vi "HFRR ADV v04.vi"() -> ()   [LabVIEW 2025] (continued)
        n290 = event-data() -> ()  [unwired: 1 in, 6 out]
        n291 = local read "Headen Service Button"() -> (w388:bool)
        n292 = case shown="True" w388 {
          frame False {
            n293 = property on="Password 3" class="Clust (strict)"("Visible"=FALSE) -> ()  [unwired: 2 in, 2 out]
            n294 = property on="Service Password Log" class="Str"("Visible"=FALSE) -> ()  [unwired: 2 in, 2 out]
          }
          frame True {
            n295 = property on="Password 3" class="Clust (strict)"("Visible"=TRUE) -> ()  [unwired: 2 in, 2 out]
            n296 = property on="Service Password Log" class="Str"("Visible"=TRUE) -> ()  [unwired: 2 in, 2 out]
          }
        }
      }
      event "Password 3.Service Password": Value Change {
        n297 = event-data() -> ()  [unwired: 1 in, 6 out]
        n298 = Unbundle By Name("Password 3") -> ("Service Password"=w395:string)
        n299 = call <vilib>:"Trim Whitespace.vi"("string"=w395) -> ("trimmed string"=w393:string)  [unwired: 1 in]
        n300 = Equal?(x=w393, y="Service@123") -> (x = y?=w394:bool)
        n301 = case shown="False" w394 {
          selector: w394 -> [w399 w401]
          frame False {
            n302 = local write "Service Password enable"(w399) -> ()
            n303 = property on="Service Password Log" class="Str"("Visible"=TRUE) -> ()  [unwired: 2 in, 2 out]
            n304 = property on="Tab Control 5" class="TabCtl (strict)"("Tabs Visible?"=TRUE ("Page Labels Display Visible?")) -> ()  [unwired: 2 in, 2 out]
          }
          frame True {
            n305 = property on="Service Password Log" class="Str"("Visible"=FALSE) -> ()  [unwired: 2 in, 2 out]
            "Service Password enable" <- w401
          }
        }
      }
      event "Sign In": Value Change {
        w403 = FALSE ("Visible")
        n306 = event-data() -> ()  [unwired: 1 in, 6 out]
        n307 = property on="About" class="Clust (strict)"("Visible"=w403) -> ()  [unwired: 2 in, 2 out]
        n308 = property on="Password 3" class="Clust (strict)"("Visible"=w403) -> ()  [unwired: 2 in, 2 out]
        n309 = property on="Service Password Log" class="Str"("Visible"=FALSE) -> ()  [unwired: 2 in, 2 out]
      }
      event "Info": Value Change {
        n310 = event-data() -> ()  [unwired: 1 in, 6 out]
        n311 = local read "Info"() -> (w405:bool)
        n312 = case shown="False" w405 {
          frame False {
            n313 = property on="About" class="Clust (strict)"("Visible"=FALSE) -> ()  [unwired: 2 in, 2 out]
          }
          frame True {
            n314 = property on="About" class="Clust (strict)"("Visible"=TRUE) -> ()  [unwired: 2 in, 2 out]
          }
        }
      }
      event "Calibration": Value Change {
        n315 = event-data() -> ()  [unwired: 1 in, 6 out]
        n316 = local read "Calibration"() -> (w409:bool)
        n317 = case shown="False" w409 {
          frame False {
            n318 = property on="Calibration 2" class="TabCtl (strict)"("Visible"=FALSE) -> ()  [unwired: 2 in, 2 out]
            n319 = local write "Cal Password"("" ("Cal Password")) -> ()
          }
          frame True {
            n320 = property on="Calibration 2" class="TabCtl (strict)"("Visible"=TRUE) -> ()  [unwired: 2 in, 2 out]
            n321 = local write "Cal Password"("" ("Cal Password")) -> ()
          }
        }
        n322 = property on="Wrong Password" class="Str"("Visible"=FALSE) -> ()  [unwired: 2 in, 2 out]
      }
      event "Cal Password": Value Change {
        n323 = event-data() -> ()  [unwired: 1 in, 6 out]
        n324 = local read "Cal Password"() -> (w417:string)
        n325 = call <vilib>:"Trim Whitespace.vi"("string"=w417) -> ("trimmed string"=w416:string)  [unwired: 1 in]
        n326 = Equal?(x=w416, y="Cal@321") -> (x = y?=w414:bool)
        n327 = case shown="True" w414 {
          frame False {
            n328 = property on="Wrong Password" class="Str"("Visible"=TRUE) -> ()  [unwired: 2 in, 2 out]
          }
          frame True {
            n329 = property on="Wrong Password" class="Str"("Visible"=FALSE) -> ()  [unwired: 2 in, 2 out]
            n330 = local write "Main Tab"(T2."About" ("Main Tab")) -> ()
            n331 = local write "Cal Password"("" ("Cal Password")) -> ()
            n332 = local write "Main Dashboard Buttons"(T1."About" ("Main Dashboard Buttons")) -> ()
            n333 = local write "Tab Control 5"(T7."Temperature Calibration" ("Tab Control 5")) -> ()
            n334 = property on="Calibration 2" class="TabCtl (strict)"("Visible"=FALSE) -> ()  [unwired: 2 in, 2 out]
            n335 = property on="Tab Control 5" class="TabCtl (strict)"("Tabs Visible?"=FALSE ("Page Labels Display Visible?")) -> ()  [unwired: 2 in, 2 out]
            n336 = local write "Calibration"(FALSE ("Calibration")) -> ()
          }
        }
      }
      event "Quit": Value Change {
        n337 = event-data() -> ()  [unwired: 1 in, 6 out]
      }
    }
    n338 = Wait (ms)(milliseconds to wait=u32 100) -> ()  [unwired: 1 out]
  }
  n339 = local write "Auto stop temp"(w12) -> ()
  n340 = local write "main tab sub"(enum32{"Page 1", "Page 2"}."Page 1" ("main tab sub")) -> ()
  n341 = local write "USERNAME"(w31) -> ()
  n342 = local write "Main Tab"(T2."HOME" ("Main Tab")) -> ()
  n343 = local write "USER ID"(w31) -> ()
  n344 = property on="Auto Scar Check  2" class="Clust (strict)"("Visible"=w12) -> (error out=w16:errorcluster)  [unwired: 2 in, 1 out]
  n345 = property on="Quit" class="Bool (strict)"("Value"=FALSE ("Quit")) -> (error out=w33:errorcluster)  [unwired: 2 in, 1 out]
  n346 = while {
    shift-right: [w429] -> _
    shift-left: "Enum - Selector" -> [w430]
    stop <- w431 stop-if-true
    # "Auto Start Logic Loop"
    n347 = case shown="\"Humidity & Temperature On\"" w430 {
      tunnel: [w434 w440 w458 w490 w521 Auto_Start_enum."Exit" ("Enum - Selector") Auto_Start_enum."Init" ("Enum - Selector")] -> w429
      frame "Init", Default {
        n348 = local read "Auto Start Test"() -> (w433:bool)
        n349 = Select(t=Auto_Start_enum."Humidity & Temperature On" ("Enum - Selector"), s=w433, f=Auto_Start_enum."Init") -> (s? t:f=w434:T10)
      }
      frame "Humidity & Temperature On" {
        n350 = flat-sequence {
          tunnel: [Auto_Start_enum."Reach point" ("Enum - Selector")] -> w437
          frame #0 {
            w441 = T13."Disabled and Grayed Out" ("Disabled")
            w442 = TRUE ("Heater Button")
            n351 = local write "Heater Button"(w442) -> ()
            n352 = local write "Humidity"(w442) -> ()
            n353 = property on="Humidity" class="Bool (strict)"("DisabledEnum"=w441) -> ()  [unwired: 2 in, 2 out]
            n354 = property on="Heater Button" class="Bool (strict)"("DisabledEnum"=w441) -> ()  [unwired: 2 in, 2 out]
          }
          frame #1 {
            n355 = local read "Set Temp"() -> (w446:dbl)
            n356 = Number To Fractional String(number=w446, precision (6)=i16 2) -> (F-format string=w445:string)  [unwired: 2 in]
            n357 = Concatenate Strings("ST;", w445) -> (w443:string)
            n358 = local write "Command"(w443) -> ()
          }
          frame #2 {
            n359 = Wait (ms)(milliseconds to wait=u32 1500) -> ()  [unwired: 1 out]
          }
          frame #3 {
            n360 = local write "Command"("HE;1" ("Command")) -> ()
          }
          frame #4 {
            n361 = Wait (ms)(milliseconds to wait=u32 1500) -> ()  [unwired: 1 out]
          }
          frame #5 {
            w451 = TRUE ("Reach point temp")
            n362 = local write "Reach point Humidity"(w451) -> ()
            n363 = local write "Reach point temp"(w451) -> ()
          }
        }
        n364 = local read "Auto Start Test"() -> (w439:bool)
        n365 = Not(x=w439) -> (.not. x?=w438:bool)
        n366 = Select(t=Auto_Start_enum."close", s=w438, f=w437) -> (s? t:f=w440:T10)
      }
      frame "Reach point" {
        w459 = TRUE ("PAUSE")
        w467 = 1.0 ("y")
        w470 = 1.0 ("y")
        n367 = local read "Set Temperature:"() -> (w471:dbl)
        n368 = local read "Set Humidity:"() -> (w466:dbl)
        n369 = local read "Humidity ( %RH )"() -> (w472:dbl)
        n370 = Add(x=w471, y=w470) -> (x+y=w469:dbl)
        n371 = Subtract(x=w471, y=w470) -> (x-y=w468:dbl)
        n372 = Add(x=w466, y=w467) -> (x+y=w465:dbl)
        n373 = Subtract(x=w466, y=w467) -> (x-y=w464:dbl)
        n374 = local read "TEMP"() -> (w473:dbl)
        n375 = In Range and Coerce(upper limit=w465, x=w472, lower limit=w464) -> (In Range?=w453:bool)  [unwired: 1 out]
        n376 = In Range and Coerce(upper limit=w469, x=w473, lower limit=w468) -> (In Range?=w454:bool)  [unwired: 1 out]
        n377 = case shown="True" w453 {
          frame False {
          }
          frame True {
            n378 = case shown="True" "Reach point Humidity" {
              selector: "Reach point Humidity" -> [_ w479]
              frame False {
              }
              frame True {
                n379 = local read "EVENT LOG"() -> (w476:string)
                n380 = Not(x=w479) -> (.not. x?=w478:bool)
                n381 = local write "Reach point Humidity"(w478) -> ()
                n382 = call "Event Log.vi"("Content"="Target Humidity reached", "EVENT LOG"=w476) -> ("EVENT LOG"=w477:string)  [unwired: 8 in, 1 out]
                n383 = local write "EVENT LOG"(w477) -> ()
              }
            }
          }
        }
        n384 = case shown="True" w454 {
          frame False {
          }
          frame True {
            n385 = case shown="True" "Reach point temp" {
              selector: "Reach point temp" -> [_ w485]
              frame False {
              }
              frame True {
                n386 = local read "EVENT LOG"() -> (w482:string)
                n387 = Not(x=w485) -> (.not. x?=w484:bool)
                n388 = local write "Reach point temp"(w484) -> ()
                n389 = call "Event Log.vi"("Content"="Target Temperature reached", "EVENT LOG"=w482) -> ("EVENT LOG"=w483:string)  [unwired: 8 in, 1 out]
                n390 = local write "EVENT LOG"(w483) -> ()
              }
            }
          }
        }
        n391 = local read "Auto Start Test"() -> (w457:bool)
        n392 = And(x=w454, y=w453) -> (x .and. y?=w463:bool)
        n393 = Select(t=Auto_Start_enum."Maintain Stage" ("Enum - Selector"), s=w463, f=Auto_Start_enum."Reach point" ("Enum - Selector")) -> (s? t:f=w460:T10)
        n394 = Not(x=w457) -> (.not. x?=w456:bool)
        n395 = Select(t=Auto_Start_enum."close", s=w456, f=w460) -> (s? t:f=w458:T10)
        n396 = call "ELAPSED TIMER VI.vi"("RESET"=w459, "PAUSE"=w459) -> ()  [unwired: 7 in, 3 out]
      }
      frame "Maintain Stage" {
        w499 = 2.0 ("y")
        w498 = 1.0 ("y")
        # "Humidity and  temperatures Set Point  have been reached"
        n397 = local read "Set Temperature:"() -> (w505:dbl)
        n398 = local read "Set Humidity:"() -> (w502:dbl)
        n399 = local read "Humidity ( %RH )"() -> (w506:dbl)
        n400 = Add(x=w505, y=w498) -> (x+y=w504:dbl)
        n401 = Subtract(x=w505, y=w498) -> (x-y=w503:dbl)
        n402 = local read "TEMP"() -> (w507:dbl)
        n403 = Add(x=w502, y=w499) -> (x+y=w501:dbl)
        n404 = Subtract(x=w502, y=w499) -> (x-y=w500:dbl)
        n405 = In Range and Coerce(upper limit=w504, x=w507, lower limit=w503) -> (In Range?=w497:bool)  [unwired: 1 out]
        n406 = In Range and Coerce(upper limit=w501, x=w506, lower limit=w500) -> (In Range?=w496:bool)  [unwired: 1 out]
        n407 = And(x=w497, y=w496) -> (x .and. y?=w495:bool)
        n408 = Not(x=w495) -> (.not. x?=w494:bool)
        n409 = call "ELAPSED TIMER VI.vi"("TARGET"=60.0, "RESET"=w494, "PAUSE"=FALSE) -> ("ELAPSED INDICATION"=w491:bool)  [unwired: 6 in, 2 out]
        n410 = case shown="True" w491 {
          tunnel: w491 -> [_ w510]
          tunnel: [Auto_Start_enum."Maintain Stage" ("Enum - Selector") w509] -> w489
          frame False {
          }
          frame True {
            n411 = stacked-sequence {
              tunnel: w510 -> [_ _ _ _ _]
              tunnel: [_ _ _ _ Auto_Start_enum."Start Stage" ("Enum - Selector")] -> w509
              frame #0 {
                n412 = local read "EVENT LOG"() -> (w512:string)
                n413 = call "Event Log.vi"("Content"="Humidity and temperature set point has stabilized.", "EVENT LOG"=w512) -> ("EVENT LOG"=w513:string)  [unwired: 8 in, 1 out]
                n414 = local write "EVENT LOG"(w513) -> ()
              }
              frame #1 {
                n415 = Wait (ms)(milliseconds to wait=u32 100) -> ()  [unwired: 1 out]
              }
              frame #2 {
                n416 = local read "EVENT LOG"() -> (w516:string)
                n417 = call "Event Log.vi"("Content"="Auto Test Started", "EVENT LOG"=w516) -> ("EVENT LOG"=w517:string)  [unwired: 8 in, 1 out]
                n418 = local write "EVENT LOG"(w517) -> ()
              }
              frame #3 {
                w518 = TRUE ("RUN")
                n419 = local write "RUN"(w518) -> ()
                "Auto Start Temp" <- w518
              }
              frame #4 {
              }
            }
          }
        }
        n420 = local read "Auto Start Test"() -> (w488:bool)
        n421 = Not(x=w488) -> (.not. x?=w487:bool)
        n422 = Select(t=Auto_Start_enum."close", s=w487, f=w489) -> (s? t:f=w490:T10)
      }
      frame "Start Stage" {
        w520 = TRUE ("PAUSE")
        n423 = local read "Auto Start Test"() -> (w525:bool)
        n424 = Not(x=w525) -> (.not. x?=w524:bool)
        n425 = Select(t=Auto_Start_enum."close" ("Enum - Selector"), s=w524, f=Auto_Start_enum."Start Stage" ("Enum - Selector")) -> (s? t:f=w521:T10)
        n426 = call "ELAPSED TIMER VI.vi"("RESET"=w520, "PAUSE"=w520) -> ()  [unwired: 7 in, 3 out]
      }
      frame "close" {
        w526 = FALSE ("Heater Button")
        n427 = local write "RUN"(w526) -> ()
        n428 = local write "Heater Button"(w526) -> ()
        n429 = local write "Humidity"(w526) -> ()
        n430 = local write "Auto Start Test"(w526) -> ()
      }
      frame "Exit" {
      }
    }
    n431 = Wait (ms)(milliseconds to wait=u32 100) -> ()  [unwired: 1 out]
    n432 = local read "Quit"() -> (w431:bool)
  }
  n433 = while {
    stop <- w555 stop-if-true
    w538 = errorcluster {"status"=FALSE, "code"=0, "source"=""} ("error in (no error) 3")
    # "this loop is for manual report generation"
    n434 = local read "Confirm Measrurement"() -> (w537:bool)
    n435 = case shown="True" w537 {
      selector: w537 -> [_ w645]
      tunnel: errorcluster {"status"=FALSE, "code"=0, "source"=""} ("error in (no error) 3") -> [_ w646]
      tunnel: [_ w644] -> _
      frame False {
      }
      frame True {
        n436 = stacked-sequence {
          tunnel: w646 -> [_ w679 _]
          tunnel: w645 -> [_ _ w786]
          tunnel: [_ w667 _] -> w644
          frame #0 {
            n437 = String To Path(string="C:\\LAB-IQ\\Image Calibrate v01.dcf") -> (path=w649:path)
            n438 = Open/Create/Replace File ("Open File")(file path (use dialog)=w649) -> (refnum out=w650:refnum<file>)  [unwired: 5 in, 2 out]
            n439 = for {
              N: 4 -> [_]
              tunnel: w650 -> [w656]
              i -> [w652]
              n440 = Read from Text File ("Read File")(file (use dialog)=w656) -> (text=w657:string)  [unwired: 3 in, 3 out]
              n441 = String Subset(string=w657, offset (0)=6, length (rest)=10 ("length (rest)")) -> (substring=w653:string)
              n442 = Fract/Exp String To Number(string=w653) -> (number=w651:dbl)  [unwired: 3 in, 1 out]
              n443 = case shown="3" w652 {
                tunnel: w651 -> [w658 w659 _ w660 _]
                frame 0 {
                  n444 = local write "5x Gain"(w658) -> ()
                }
                frame 1 {
                  n445 = local write "10x Gain"(w659) -> ()
                }
                frame 2 {
                }
                frame 3 {
                  n446 = local write "100x gain"(w660) -> ()
                }
                frame 4, Default {
                }
              }
            }
          }
          frame #1 {
            n447 = local read "TEST STANDARD"() -> (w662:T3)
            n448 = case shown="\"ISO 12156\"" w662 {
              tunnel: ["ASTM D6079" "ISO 12156"] -> w661
              frame "ASTM D6079", Default {
              }
              frame "ISO 12156" {
              }
            }
            n449 = call "IMAGE ANALYSIS.vi"("Enum"=POST_ANALYSIS_ENUM."GET MEASUREMENTS", "error in"=w679) -> ("error out"=w686:errorcluster)  [unwired: 8 in, 1 out]
            n450 = local read "Magnification :"() -> (w672:string)
            n451 = call "Stall Data Flow.vim"("value in"=w686, "milliseconds to wait"=u32 1000) -> ("value out"=w685:errorcluster)  [unwired: 1 out]
            n452 = local read "Test File List :"() -> (w683:string)
            n453 = case shown="\"10x\"" w672 {
              tunnel: [w722 w723] -> w670
              frame "5x", Default {
                n454 = local read "5x Gain"() -> (w722:dbl)
              }
              frame "10x" {
                # "5x"
                n455 = local read "10x Gain"() -> (w723:dbl)
              }
            }
            n456 = call "IMAGE ANALYSIS.vi"("Enum"=POST_ANALYSIS_ENUM."READ", "error in"=w685) -> ("error out"=w682:errorcluster, "data out"=w673:string)  [unwired: 8 in]
            n457 = Match Pattern(string=w673, regular expression="\"type\": ") -> (after substring=w677:string)  [unwired: 1 in, 3 out]
            n458 = call "IMAGE PATH CREATION PY.vi"("error in (no error)"=w682, "File Name :"=w683) -> ("error out"=w681:errorcluster, "File Path"=w669:path, "File Path String:"=w664:string)  [unwired: 7 in]
            n459 = Match Pattern(string=w677, regular expression=",") -> (before substring=w663:string)  [unwired: 1 in, 3 out]
            n460 = local read "Calibration Tab"() -> (w666:enum32{"Measrument", "Calibrate"})
            n461 = call "Stall Data Flow.vim"("value in"=w681, "milliseconds to wait"=u32 250) -> ("value out"=w665:errorcluster)  [unwired: 1 out]
            n462 = Equal?(x=w663, y="\"rectangle\"") -> (x = y?=w674:bool)
            n463 = case shown="False" w674 {
              tunnel: w673 -> [w728 w783]
              tunnel: w670 -> [_ w774]
              tunnel: cluster{"major":dbl, "minor":dbl, "average":dbl} {"major"=0.0, "minor"=0.0, "average"=0.0} -> [w726 w770]
              tunnel: [w725 w767] -> w668
              tunnel: w663 -> [w727 _]
              tunnel: w670 -> [w724 _]
              frame False {
                n464 = Equal?(x=w727, y="\"line\"") -> (x = y?=w729:bool)
                n465 = case shown="True" w729 {
                  tunnel: w728 -> [_ w744]
                  tunnel: w726 -> [w731 w743]
                  tunnel: [w731 w741] -> w725
                  tunnel: w724 -> [_ w740]
                  frame False {
                  }
                  frame True {
                    w739 = 0.0 ("Major Axis")
                    n466 = Match Pattern(string=w744, regular expression="\"length_px\":") -> (after substring=w742:string)  [unwired: 1 in, 3 out]
                    n467 = property on="Major Axis" class="DigNum (strict)"("Caption.Text"="") -> ()  [unwired: 2 in, 2 out]
                    n468 = property on="Minor Axis" class="DigNum (strict)"("Caption.Text"="") -> ()  [unwired: 2 in, 2 out]
                    n469 = property on="Average" class="DigNum (strict)"("Caption.Text"="Line") -> ()  [unwired: 2 in, 2 out]
                    n470 = Fract/Exp String To Number(string=w742, default (0 dbl)=0.0 ("default (0 DBL)")) -> (number=w738:dbl)  [unwired: 2 in, 1 out]
                    "Pixel Value" <- w738
                    n471 = Multiply(x=w738, y=w740) -> (x*y=w751:dbl)
                    n472 = Multiply(x=w751, y=1000.0) -> (x*y=w734:dbl)
                    n473 = Divide(x=w734, y=1000.0) -> (x/y=w737:dbl)
                    n474 = local write "Measurment (mm)"(w737) -> ()
                    n475 = Bundle By Name(cluster=w743, "average"=w734) -> (w741:cluster{"major":dbl, "minor":dbl, "average":dbl})
                    n476 = Number To Fractional String(number=w734, precision (6)=i16 1) -> (F-format string=w733:string)  [unwired: 2 in]
                    n477 = local write "Minor Axis"(w739) -> ()
                    n478 = local write "Major Axis"(w739) -> ()
                    n479 = Fract/Exp String To Number(string=w733) -> (number=w732:dbl)  [unwired: 3 in, 1 out]
                    n480 = local write "Average"(w732) -> ()
                  }
                }
              }
              frame True {
                w771 = 1000.0 ("y")
                w777 = 0.0 ("default (0 DBL)")
                n481 = Match Pattern(string=w783, regular expression=" \"width_px\":") -> (after substring=w781:string)  [unwired: 1 in, 3 out]
                n482 = Match Pattern(string=w781, regular expression="\"height_px\":") -> (before substring=w779:string, after substring=w778:string)  [unwired: 1 in, 2 out]
                n483 = Fract/Exp String To Number(string=w779, default (0 dbl)=w777) -> (number=w776:dbl)  [unwired: 2 in, 1 out]
                n484 = Fract/Exp String To Number(string=w778, default (0 dbl)=w777) -> (number=w775:dbl)  [unwired: 2 in, 1 out]
                n485 = Multiply(x=w776, y=w774) -> (x*y=w773:dbl)
                n486 = Multiply(x=w775, y=w774) -> (x*y=w772:dbl)
                n487 = Multiply(x=w773, y=w771) -> (x*y=w757:dbl)
                n488 = Multiply(x=w772, y=w771) -> (x*y=w755:dbl)
                n489 = Add(x=w757, y=w755) -> (x+y=w769:dbl)
                n490 = property on="Major Axis" class="DigNum (strict)"("Caption.Text"="Major Axis") -> ()  [unwired: 2 in, 2 out]
                n491 = property on="Minor Axis" class="DigNum (strict)"("Caption.Text"="Minor Axis") -> ()  [unwired: 2 in, 2 out]
                n492 = property on="Average" class="DigNum (strict)"("Caption.Text"="Average") -> ()  [unwired: 2 in, 2 out]
                n493 = Divide(x=w769, y=2.0) -> (x/y=w753:dbl)
                n494 = Bundle By Name(cluster=w770, "major"=w757, "minor"=w755, "average"=w753) -> (w767:cluster{"major":dbl, "minor":dbl, "average":dbl})
                n495 = Number To Fractional String(number=w755, precision (6)=i16 1) -> (F-format string=w762:string)  [unwired: 2 in]
                n496 = Number To Fractional String(number=w753, precision (6)=i16 1) -> (F-format string=w763:string)  [unwired: 2 in]
                n497 = Number To Fractional String(number=w757, precision (6)=i16 1) -> (F-format string=w761:string)  [unwired: 2 in]
                n498 = Fract/Exp String To Number(string=w762) -> (number=w754:dbl)  [unwired: 3 in, 1 out]
                n499 = Fract/Exp String To Number(string=w763) -> (number=w752:dbl)  [unwired: 3 in, 1 out]
                n500 = Fract/Exp String To Number(string=w761) -> (number=w756:dbl)  [unwired: 3 in, 1 out]
                n501 = local write "Major Axis"(w756) -> ()
                n502 = local write "Average"(w752) -> ()
                n503 = local write "Minor Axis"(w754) -> ()
              }
            }
            n504 = case shown="\"Measrument\", Default" w666 {
              tunnel: w669 -> [w696 _]
              tunnel: w668 -> [w695 _]
              tunnel: [w692 w721] -> w667
              tunnel: w665 -> [w694 w721]
              tunnel: w664 -> [w693 _]
              tunnel: w661 -> [w691 _]
              frame "Measrument", Default {
                n505 = stacked-sequence {
                  tunnel: w696 -> [w714 _]
                  tunnel: w695 -> [w712 _]
                  tunnel: w694 -> [w710 _]
                  tunnel: w693 -> [w709 _]
                  tunnel: [w704 _] -> w692
                  tunnel: w691 -> [w697 _]
                  frame #0 {
                    n506 = call "IMAGE ANALYSIS.vi"("Enum"=POST_ANALYSIS_ENUM."SAVE IMAGE", "error in"=w710, "IMAGE FILE PATH"=w709) -> ("error out"=w708:errorcluster)  [unwired: 7 in, 1 out]
                    n507 = call "Stall Data Flow.vim"("value in"=w708, "milliseconds to wait"=u32 1000) -> ("value out"=w699:errorcluster)  [unwired: 1 out]
                    n508 = local read "Test File List :"() -> (w716:string)
                    n509 = call "IMAGE ANALYSIS.vi"("Enum"=POST_ANALYSIS_ENUM."MINIMIZE UI", "error in"=w699) -> ("error out"=w706:errorcluster)  [unwired: 8 in, 1 out]
                    n510 = Bundle By Name(cluster=T18 {"File Name"="", "Test Method"="", "Operator"="", "Fuel Description"="", "Date and time"=""} ("Main Ref"), "Test Method"=w697, "File Name"=w716) -> (w717:T18)
                    n511 = call "Stall Data Flow.vim"("value in"=w706, "milliseconds to wait"=u32 1500) -> ("value out"=w701:errorcluster)  [unwired: 1 out]
                    n512 = call "duf file read.vi"("error in (no error)"=w701, "Main Ref"=w717) -> ("error out"=w715:errorcluster, "Main Ref 2"=w713:T18)  [unwired: 8 in]
                    n513 = call "DETECTION REPORT for manual.vi"("error in (no error)"=w715, "return value 3"=w712, "Image File Path"=w714, "Main Ref"=w713) -> ("error out"=w711:errorcluster)  [unwired: 7 in]
                    n514 = call <vilib>:"Clear Errors.vi"("error in (no error)"=w711) -> ("error out"=w702:errorcluster)  [unwired: 5 in, 1 out]
                    n515 = call "IMAGE ANALYSIS.vi"("Enum"=POST_ANALYSIS_ENUM."MINIMIZE UI", "error in"=w702) -> ("error out"=w704:errorcluster)  [unwired: 8 in, 1 out]
                  }
                  frame #1 {
                    n516 = local write "Main Tab"(T2."HOME" ("Main Tab")) -> ()
                    n517 = local write "Main Dashboard Buttons"(T1."Home" ("Main Dashboard Buttons")) -> ()
                  }
                }
              }
              frame "Calibrate" {
              }
            }
          }
          frame #2 {
            n518 = Not(x=w786) -> (.not. x?=w785:bool)
            n519 = local write "Confirm Measrurement"(w785) -> ()
            n520 = local read "Calibration Tab"() -> (w784:enum32{"Measrument", "Calibrate"})
            n521 = case shown="\"Measrument\", Default" w784 {
              frame "Measrument", Default {
                n522 = local write "Main Tab"(T2."HOME" ("Main Tab")) -> ()
              }
              frame "Calibrate" {
              }
            }
          }
        }
      }
    }
    n523 = local read "Humidity"() -> (w529:bool)
    n524 = local read "Save Change"() -> (w534:bool)
    n525 = local read "Calibrate"() -> (w535:bool)
    n526 = local read "Auto Start Test"() -> (w530:bool)
    n527 = case shown="True" w535 {
      selector: w535 -> [_ w642]
      frame False {
      }
      frame True {
        n528 = Not(x=w642) -> (.not. x?=w641:bool)
        n529 = local write "Calibrate"(w641) -> ()
        n530 = local write "Calibration Tab"(enum32{"Measrument", "Calibrate"}."Calibrate" ("Calibration Tab")) -> ()
      }
    }
    n531 = case shown="True" w534 {
      selector: w534 -> [_ w586]
      frame False {
      }
      frame True {
        n532 = stacked-sequence {
          tunnel: w586 -> [_ _ _ _ w640]
          frame #0 {
            n533 = call "IMAGE ANALYSIS.vi"("Enum"=POST_ANALYSIS_ENUM."HIDE UI") -> ()  [unwired: 9 in, 2 out]
          }
          frame #1 {
            n534 = local read "100x gain"() -> (w588:dbl)
            n535 = local read "10x Gain"() -> (w589:dbl)
            n536 = local read "5x Gain"() -> (w590:dbl)
            n537 = Number To Fractional String(number=w589, width (-)=i16 4, precision (6)=i16 7) -> (F-format string=w611:string)  [unwired: 1 in]
            n538 = Number To Fractional String(number=0.0, width (-)=i16 4, precision (6)=i16 7) -> (F-format string=w606:string)  [unwired: 1 in]
            n539 = Number To Fractional String(number=w588, width (-)=i16 4, precision (6)=i16 7) -> (F-format string=w594:string)  [unwired: 1 in]
            n540 = Number To Fractional String(number=w590, width (-)=i16 10 ("precision (6)"), precision (6)=i16 7) -> (F-format string=w620:string)  [unwired: 1 in]
            n541 = Concatenate Strings("[CH1]" ("string"), w620, " - 5x Gain" ("string"), "\r") -> (w610:string)
            n542 = Concatenate Strings("[CH2]" ("string"), w611, " - 10x Gain" ("string"), "\r") -> (w609:string)
            n543 = Concatenate Strings("[CH3]" ("string"), w606, " - 20x Gain" ("string"), "\r") -> (w600:string)
            n544 = Concatenate Strings("[CH4]" ("string"), w594, " - 100x Gain" ("string"), "\r") -> (w593:string)
            n545 = String To Path(string="C:\\LAB-IQ\\Image Calibrate v01.dcf") -> (path=w623:path)
            n546 = Concatenate Strings(w610, w609, w600, w593) -> (w608:string)
            n547 = call <vilib>:"Write Characters To File.vi"("append to file? (new file:F)"=FALSE, "character string"=w608, "file path (dialog if empty)"=w623) -> ()  [unwired: 2 in, 1 out]
          }
          frame #2 {
            n548 = String To Path(string="C:\\LAB-IQ\\Image Calibrate v01.dcf") -> (path=w626:path)
            n549 = Open/Create/Replace File ("Open File")(file path (use dialog)=w626) -> (refnum out=w627:refnum<file>)  [unwired: 5 in, 2 out]
            n550 = for {
              N: 4 -> [_]
              tunnel: w627 -> [w633]
              i -> [w629]
              n551 = Read from Text File ("Read File")(file (use dialog)=w633) -> (text=w634:string)  [unwired: 3 in, 3 out]
              n552 = String Subset(string=w634, offset (0)=6, length (rest)=10 ("length (rest)")) -> (substring=w630:string)
              n553 = Fract/Exp String To Number(string=w630) -> (number=w628:dbl)  [unwired: 3 in, 1 out]
              n554 = case shown="3" w629 {
                tunnel: w628 -> [w635 w636 _ w637 _]
                frame 0 {
                  n555 = local write "5x Gain"(w635) -> ()
                }
                frame 1 {
                  n556 = local write "10x Gain"(w636) -> ()
                }
                frame 2 {
                }
                frame 3 {
                  n557 = local write "100x gain"(w637) -> ()
                }
                frame 4, Default {
                }
              }
            }
          }
          frame #3 {
            n558 = call "IMAGE ANALYSIS.vi"("Enum"=POST_ANALYSIS_ENUM."SHOW UI") -> ()  [unwired: 9 in, 2 out]
          }
          frame #4 {
            n559 = Not(x=w640) -> (.not. x?=w639:bool)
            n560 = local write "Save Change"(w639) -> ()
          }
        }
      }
    }
    n561 = case shown="False" w530 {
      tunnel: w529 -> [w556 _]
      frame False {
        n562 = case shown="True" w556 {
          frame False {
          }
          frame True {
            n563 = local read "Set Humidity:"() -> (w560:dbl)
            n564 = local read "Set Humidity:"() -> (w563:dbl)
            n565 = local read "Humidity ( %RH )"() -> (w564:dbl)
            n566 = Subtract(x=w560, y=2.0) -> (x-y=w558:dbl)
            n567 = Add(x=w563, y=2.0) -> (x+y=w559:dbl)
            n568 = In Range and Coerce(upper limit=w559, x=w564, lower limit=w558) -> (In Range?=w557:bool)  [unwired: 1 out]
            n569 = case shown="True" w557 {
              frame False {
              }
              frame True {
                n570 = case shown="False" "Manual Humididty Reached" {
                  selector: "Manual Humididty Reached" -> [_ w567]
                  frame False {
                  }
                  frame True {
                    n571 = Not(x=w567) -> (.not. x?=w566:bool)
                    n572 = local write "Manual Humididty Reached"(w566) -> ()
                    n573 = local read "EVENT LOG"() -> (w569:string)
                    n574 = call "Event Log.vi"("Content"="Target Humidity reached", "EVENT LOG"=w569) -> ("EVENT LOG"=w568:string)  [unwired: 8 in, 1 out]
                    n575 = local write "EVENT LOG"(w568) -> ()
                  }
                }
              }
            }
          }
        }
      }
      frame True {
        n576 = local write "Manual Humididty Reached"(TRUE ("Manual Humididty Reached")) -> ()
      }
    }
    n577 = local read "Cap Live Image"() -> (w550:bool)
    n578 = local read "SCAR MEASURMENT"() -> (w553:enum32{"Auto Scar", "Manual Scar"})
    n579 = Wait (ms)(milliseconds to wait=u32 250) -> ()  [unwired: 1 out]
    n580 = Equal?(x=w553, y=enum32{"Auto Scar", "Manual Scar"}."Manual Scar" ("SCAR MEASURMENT")) -> (x = y?=w551:bool)
    n581 = And(x=w551, y=w550) -> (x .and. y?=w549:bool)
    n582 = case shown="True" w549 {
      selector: w549 -> [_ w865]
      frame False {
      }
      frame True {
        n583 = stacked-sequence {
          tunnel: [_ _ _ w880 _] -> _
          tunnel: w865 -> [_ _ _ _ w886]
          frame #0 {
            w866 = 0.0
            n584 = local write "Major Axis"(w866) -> ()
            n585 = local write "Minor Axis"(w866) -> ()
            n586 = local write "Average"(w866) -> ()
          }
          frame #1 {
            n587 = call "CAMERA LIVE FEED FGV.vi"("Enum - Menu"=CAMERA_LIVE_FEED_ENUM."CAMERA MINIMIZE") -> ()  [unwired: 9 in, 2 out]
          }
          frame #2 {
            n588 = local read "FILE 3"() -> (w874:string)
            n589 = call <vilib>:"Trim Whitespace.vi"("string"="C:\\LAB-IQ\\images\\") -> ("trimmed string"=w876:string)  [unwired: 1 in]
            n590 = String To Path(string=w876) -> (path=w875:path)
            n591 = Concatenate Strings(w874, ".png" ("string")) -> (w873:string)
            n592 = Build Path(base path=w875, name or relative path=w873) -> (appended path=w871:path)
            n593 = Path To String(path=w871) -> (string=w870:string)
            n594 = call "CAMERA LIVE FEED FGV.vi"("Enum - Menu"=CAMERA_LIVE_FEED_ENUM."CAMERA SAVE", "Image Path"=w870) -> ("error out"=w868:errorcluster)  [unwired: 8 in, 1 out]
            n595 = case shown="No Error" w868 {
              frame No Error {
                n596 = One Button Dialog(message="Image saved successfully") -> ()  [unwired: 1 in, 1 out]
              }
              frame Error {
              }
            }
          }
          frame #3 {
            n597 = call "LIST FILE NAMES.vi"() -> ("error out"=w882:errorcluster, "filenames"=w879:string[])  [unwired: 10 in]
            n598 = call "IMAGE ANALYSIS.vi"("Enum"=POST_ANALYSIS_ENUM."SHOW UI", "error in"=w882) -> ("error out"=w880:errorcluster)  [unwired: 8 in, 1 out]
            n599 = property on="Test File List :" class="CmbBox"("Strings[]"=w879) -> ()  [unwired: 2 in, 2 out]
          }
          frame #4 {
            (unwired) T19."Report" ("Main Dashboard Buttons")
            n600 = Not(x=w886) -> (.not. x?=w885:bool)
            n601 = local write "Zoom Factore"(0.0 ("Zoom Factore")) -> ()
            n602 = local write "Cap Live Image"(w885) -> ()
            n603 = local write "Main Tab"(T2."Adv Scar Report" ("Main Tab")) -> ()
            n604 = property on="Cap Live Image" class="Bool (strict)"("BoolText.Text"="Capture Image" ("Boolean Text.Text")) -> ()  [unwired: 2 in, 2 out]
            n605 = local write "Main Dashboard Buttons"(T1."Report" ("Main Dashboard Buttons")) -> ()
          }
        }
      }
    }
    n606 = local read "change Gain"() -> (w533:bool)
    n607 = local read "Back Square"() -> (w532:bool)
    n608 = case shown="True" w533 {
      selector: w533 -> [_ w577]
      frame False {
      }
      frame True {
        n609 = stacked-sequence {
          tunnel: w577 -> [_ w585]
          frame #0 {
            n610 = local read "Actual (µm)"() -> (w581:dbl)
            n611 = local read "Pixel Value"() -> (w580:dbl)
            n612 = local read "Magnification :"() -> (w579:string)
            n613 = Divide(x=w581, y=w580) -> (x/y=w578:dbl)
            n614 = case shown="\"10x\"" w579 {
              tunnel: w578 -> [w582 w583]
              frame "10x" {
                n615 = local write "10x Gain"(w582) -> ()
              }
              frame "5x", Default {
                n616 = local write "5x Gain"(w583) -> ()
              }
            }
          }
          frame #1 {
            n617 = Not(x=w585) -> (.not. x?=w584:bool)
            n618 = local write "change Gain"(w584) -> ()
          }
        }
      }
    }
    n619 = case shown="True" w532 {
      selector: w532 -> [_ w575]
      frame False {
      }
      frame True {
        n620 = Not(x=w575) -> (.not. x?=w574:bool)
        n621 = local write "Back Square"(w574) -> ()
        n622 = local write "Calibration Tab"(enum32{"Measrument", "Calibrate"}."Measrument" ("Calibration Tab")) -> ()
      }
    }
    n623 = local read "Rectangle Tool"() -> (w544:bool)
    n624 = local read "Clear ROI Tool"() -> (w543:bool)
    n625 = local read "Open Image"() -> (w548:bool)
    n626 = local read "line tool"() -> (w545:bool)
    n627 = local read "OUT"() -> (w546:bool)
    n628 = local read "In"() -> (w547:bool)
    n629 = case shown="True" w548 {
      selector: w548 -> [_ w853]
      tunnel: [w849 w855] -> _
      tunnel: w538 -> [w849 w854]
      frame False {
      }
      frame True {
        n630 = Not(x=w853) -> (.not. x?=w852:bool)
        n631 = local write "Open Image"(w852) -> ()
        n632 = call "IMAGE ANALYSIS.vi"("Enum"=POST_ANALYSIS_ENUM."HIDE UI", "error in"=w854) -> ("error out"=w862:errorcluster)  [unwired: 8 in, 1 out]
        n633 = call "File Dialog"("start path"=path "C:/LAB-IQ/images", "error in"=w862) -> ("selected path"=w851:path, "error out"=w860:errorcluster)  [unwired: 10 in, 2 out]
        "Image path  2" <- w851
        n634 = call <vilib>:"Clear Errors.vi"("error in (no error)"=w860) -> ("error out"=w859:errorcluster)  [unwired: 5 in, 1 out]
        n635 = call "IMAGE ANALYSIS.vi"("Enum"=POST_ANALYSIS_ENUM."OPEN FILE", "error in"=w859, "File Path"=w851) -> ("error out"=w858:errorcluster)  [unwired: 7 in, 1 out]
        n636 = call <vilib>:"Clear Errors.vi"("error in (no error)"=w858) -> ("error out"=w857:errorcluster)  [unwired: 5 in, 1 out]
        n637 = call "IMAGE ANALYSIS.vi"("Enum"=POST_ANALYSIS_ENUM."SHOW UI", "error in"=w857) -> ("error out"=w855:errorcluster)  [unwired: 8 in, 1 out]
        n638 = local write "Zoom Factore"(100.0 ("Zoom Factore")) -> ()
      }
    }
    n639 = case shown="True" w546 {
      selector: w546 -> [_ w834]
      tunnel: w538 -> [w831 w839]
      tunnel: [w831 w833] -> _
      frame False {
      }
      frame True {
        n640 = Not(x=w834) -> (.not. x?=w832:bool)
        n641 = local read "Zoom Factore"() -> (w837:dbl)
        n642 = local write "OUT"(w832) -> ()
        n643 = call "IMAGE ANALYSIS.vi"("Enum"=POST_ANALYSIS_ENUM."ZOOM OUT", "error in"=w839) -> ("error out"=w833:errorcluster)  [unwired: 8 in, 1 out]
        n644 = Divide(x=w837, y=1.2) -> (x/y=w835:dbl)
        n645 = local write "Zoom Factore"(w835) -> ()
      }
    }
    n646 = case shown="True" w547 {
      selector: w547 -> [_ w843]
      tunnel: w538 -> [w840 w848]
      tunnel: [w840 w841] -> _
      frame False {
      }
      frame True {
        n647 = Not(x=w843) -> (.not. x?=w842:bool)
        n648 = local read "Zoom Factore"() -> (w846:dbl)
        n649 = local write "In"(w842) -> ()
        n650 = call "IMAGE ANALYSIS.vi"("Enum"=POST_ANALYSIS_ENUM."ZOOM IN", "error in"=w848) -> ("error out"=w841:errorcluster)  [unwired: 8 in, 1 out]
        n651 = Multiply(x=w846, y=1.2) -> (x*y=w844:dbl)
        n652 = local write "Zoom Factore"(w844) -> ()
      }
    }
    n653 = case shown="True" w543 {
      selector: w543 -> [_ w815]
      tunnel: w538 -> [w813 w817]
      tunnel: [w813 w816] -> _
      frame False {
      }
      frame True {
        n654 = Not(x=w815) -> (.not. x?=w814:bool)
        n655 = local write "Clear ROI Tool"(w814) -> ()
        n656 = call "IMAGE ANALYSIS.vi"("Enum"=POST_ANALYSIS_ENUM."CLEAR ROI", "error in"=w817) -> ("error out"=w816:errorcluster)  [unwired: 8 in, 1 out]
      }
    }
    n657 = case shown="True" w545 {
      selector: w545 -> [_ w827]
      tunnel: w538 -> [w825 w830]
      tunnel: [w825 w828] -> _
      frame False {
      }
      frame True {
        n658 = Not(x=w827) -> (.not. x?=w826:bool)
        n659 = local write "line tool"(w826) -> ()
        n660 = call "IMAGE ANALYSIS.vi"("Enum"=POST_ANALYSIS_ENUM."DRAW LINE", "error in"=w830) -> ("error out"=w828:errorcluster)  [unwired: 8 in, 1 out]
      }
    }
    n661 = case shown="True" w544 {
      selector: w544 -> [_ w821]
      tunnel: w538 -> [w819 w823]
      tunnel: [w819 w822] -> _
      frame False {
      }
      frame True {
        n662 = Not(x=w821) -> (.not. x?=w820:bool)
        n663 = local write "Rectangle Tool"(w820) -> ()
        n664 = call "IMAGE ANALYSIS.vi"("Enum"=POST_ANALYSIS_ENUM."DRAW REC", "error in"=w823) -> ("error out"=w822:errorcluster)  [unwired: 8 in, 1 out]
      }
    }
    n665 = local read "SCAR MEASURMENT"() -> (w531:enum32{"Auto Scar", "Manual Scar"})
    n666 = local read "Fit to Screen Tool"() -> (w540:bool)
    n667 = local read "Resize Tool"() -> (w539:bool)
    n668 = case shown="\"Manual Scar\", Default" w531 {
      frame "Auto Scar" {
        n669 = property on="Cap Live Image" class="Bool (strict)"("BoolText.Text"="Report" ("Boolean Text.Text")) -> ()  [unwired: 2 in, 2 out]
      }
      frame "Manual Scar", Default {
        n670 = property on="Cap Live Image" class="Bool (strict)"("BoolText.Text"="Save Image" ("Boolean Text.Text")) -> ()  [unwired: 2 in, 2 out]
      }
    }
    n671 = local read "ROI Color Tool"() -> (w541:bool)
    n672 = local read "Pan Tool"() -> (w542:bool)
    n673 = case shown="True" w542 {
      selector: w542 -> [_ w809]
      tunnel: w538 -> [w807 w811]
      tunnel: [w807 w810] -> _
      frame False {
      }
      frame True {
        n674 = Not(x=w809) -> (.not. x?=w808:bool)
        n675 = call "IMAGE ANALYSIS.vi"("Enum"=POST_ANALYSIS_ENUM."PAN", "error in"=w811) -> ("error out"=w810:errorcluster)  [unwired: 8 in, 1 out]
        n676 = local write "Pan Tool"(w808) -> ()
      }
    }
    n677 = case shown="True" w539 {
      selector: w539 -> [_ w793]
      tunnel: w538 -> [w788 w790]
      tunnel: [w788 w789] -> _
      frame False {
      }
      frame True {
        n678 = Not(x=w793) -> (.not. x?=w792:bool)
        n679 = local write "Resize Tool"(w792) -> ()
        n680 = call "IMAGE ANALYSIS.vi"("Enum"=POST_ANALYSIS_ENUM."RESIZE MODE", "error in"=w790) -> ("error out"=w789:errorcluster)  [unwired: 8 in, 1 out]
      }
    }
    n681 = case shown="True" w540 {
      selector: w540 -> [_ w798]
      tunnel: [w794 w799] -> _
      tunnel: w538 -> [w794 w797]
      frame False {
      }
      frame True {
        n682 = Not(x=w798) -> (.not. x?=w796:bool)
        n683 = local write "Zoom Factore"(100.0 ("Zoom Factore")) -> ()
        n684 = local write "Fit to Screen Tool"(w796) -> ()
        n685 = call "IMAGE ANALYSIS.vi"("Enum"=POST_ANALYSIS_ENUM."FIT", "error in"=w797) -> ("error out"=w799:errorcluster)  [unwired: 8 in, 1 out]
      }
    }
    n686 = case shown="True" w541 {
      selector: w541 -> [_ w804]
      tunnel: [w801 w805] -> _
      tunnel: w538 -> [w801 w802]
      frame False {
      }
      frame True {
        n687 = Not(x=w804) -> (.not. x?=w803:bool)
        n688 = local write "ROI Color Tool"(w803) -> ()
        n689 = call "IMAGE ANALYSIS.vi"("Enum"=POST_ANALYSIS_ENUM."SET ROI COLOR", "error in"=w802) -> ("error out"=w805:errorcluster)  [unwired: 8 in, 1 out]
      }
    }
    n690 = local read "Quit"() -> (w555:bool)
  }
  n691 = property on="Service Password Log" class="Str"("Visible"=w12) -> ()  [unwired: 2 in, 2 out]
  n692 = property on="Password 3" class="Clust (strict)"("Visible"=w12) -> ()  [unwired: 2 in, 2 out]
  n693 = while {
    stop <- w889 stop-if-true
    n694 = local read "Image Path"() -> (w892:path)
    n695 = local read "Print 3"() -> (w895:bool)
    n696 = Equal?(x=w892, y=path "") -> (x = y?=w891:bool)
    n697 = Not(x=w891) -> (.not. x?=w890:bool)
    n698 = property on="Print 3" class="Bool (strict)"("Visible"=w890) -> ()  [unwired: 2 in, 2 out]
    n699 = case shown="True" w895 {
      frame False {
        n700 = local write "Rd"(TRUE ("Boolean 7")) -> ()
      }
      frame True {
        n701 = flat-sequence {
          tunnel: [w935] -> w903
          tunnel: [w922] -> w901
          tunnel: [w932] -> w897
          tunnel: w903 -> [w944]
          tunnel: [w944] -> w902
          tunnel: w901 -> [w943]
          tunnel: [w943] -> w900
          tunnel: [w941] -> w899
          tunnel: [w940] -> w898
          tunnel: w897 -> [w940]
          tunnel: w902 -> [w946]
          tunnel: w900 -> [w947]
          tunnel: w899 -> [_]
          tunnel: w898 -> [w945]
          frame #0 {
            n702 = case shown="True" "Rd" {
              frame False {
              }
              frame True {
                n703 = while {
                  tunnel: "abcdefABCDEF" ("string 2") -> [w914]
                  shift-right: [w912] -> w906
                  shift-left: "" -> [w911]
                  i -> [w921]
                  stop <- w920 stop-if-true
                  n704 = Random Number (0-1)() -> (number: 0 to 1=w915:dbl)
                  n705 = Multiply(x=w915, y=62.0) -> (x*y=w917:dbl)
                  n706 = Decrement(x="Length 2") -> (x-1=w910:i16)
                  n707 = To Word Integer(number=w917) -> (16bit integer=w918:i16)
                  n708 = String Subset(string=w914, offset (0)=w918, length (rest)=1 ("length (rest)")) -> (substring=w913:string)
                  n709 = Greater Or Equal?(x=w921, y=w910) -> (x >= y?=w920:bool)
                  n710 = Concatenate Strings(w913, w911) -> (w912:string)
                }
                "String 10" <- w906
                n711 = local write "Rd"(FALSE ("Boolean 7")) -> ()
              }
            }
          }
          frame #1 {
            w933 = "_resized.jpg" ("command line")
            (unwired) ".jpg -resize 320x240 " ("string")
            (unwired) "Choose an Image File" ("prompt")
            # "-resize 1798x425"
            n712 = local read "Image Path"() -> (w927:path)
            n713 = Strip Path(path=w927) -> (stripped path=w922:path, name=w923:string)
            n714 = Match Pattern(string=w923, regular expression=".jpg") -> (before substring=→"before substring 2":string, after substring=→"after substring":string)  [unwired: 1 in, 2 out]
            n715 = Match Pattern(string=w923, regular expression="\\") -> (before substring=w929:string)  [unwired: 1 in, 3 out]
            n716 = Match Pattern(string=w929, regular expression=".jpg") -> (before substring=w928:string)  [unwired: 1 in, 3 out]
            n717 = Concatenate Strings("cmd /c convert " ("string"), w928, ".jpg -resize 320x240  " ("command line"), w928, w933) -> (w936:string)
            n718 = call <vilib>:"System Exec.vi"("run minimized? (F)"=TRUE, "wait until completion? (T)"=TRUE, "working directory"=w922, "command line"=w936) -> ("error out"=w935:errorcluster)  [unwired: 4 in, 3 out]
            "error out 2" <- w935
            n719 = Concatenate Strings(w928, w933) -> (w932:string)
          }
          frame #2 {
            n720 = Wait (ms)(milliseconds to wait=u32 2000 ("millisecond timer value")) -> (millisecond timer value=w941:u32)
          }
          frame #3 {
            n721 = case shown="No Error" w946 {
              tunnel: w947 -> [w950 _]
              tunnel: w945 -> [w948 _]
              frame No Error {
                (unwired) ".jpg" ("string")
                n722 = Path To String(path=w950) -> (string=w954:string)
                n723 = Concatenate Strings(w954, "\\" ("string"), w948) -> (w953:string)
                n724 = String To Path(string=w953) -> (path=w952:path)
                n725 = call <vilib>:"Read JPEG File.vi"("path to JPEG file"=w952) -> ("image data"=w956:T11)  [unwired: 8 in, 2 out]
                "image data" <- w956
                n726 = local write "Print 3"(FALSE ("Print 2")) -> ()
                n727 = call <vilib>:"Draw Flattened Pixmap.vi"("image data"=w956) -> ("new picture"=→"new picture":picture)  [unwired: 8 in]
              }
              frame Error {
              }
            }
          }
        }
      }
    }
    n728 = Wait (ms)(milliseconds to wait=u32 20 ("millisecond timer value")) -> ()  [unwired: 1 out]
    n729 = local read "Quit"() -> (w889:bool)
  }
  n730 = while {
    tunnel: w33 -> [_]
    tunnel: w16 -> [_]
    stop <- w987 stop-if-true
    # "New Adv Logics"
    n731 = local read "Main Tab"() -> (w966:T2)
    n732 = local read "Main Tab"() -> (w985:T2)
    n733 = local read "Sign In"() -> (w984:bool)
    n734 = case shown="\"Adv Scar\"" w966 {
      frame "HOME", Default {
        n735 = local read "LIVE FEED MIN TEMP"() -> (w1114:bool)
        n736 = local write "LIVE FEED MAX TEMP"(TRUE ("LIVE FEED MAX TEMP")) -> ()
        n737 = local read "CAMERA ROI MIN TEMP"() -> (w1112:bool)
        n738 = case shown="True" w1114 {
          selector: w1114 -> [_ w1121]
          frame False {
          }
          frame True {
            n739 = Not(x=w1121) -> (.not. x?=w1120:bool)
            n740 = local write "LIVE FEED MIN TEMP"(w1120) -> ()
            n741 = call "CAMERA LIVE FEED FGV.vi"("Enum - Menu"=CAMERA_LIVE_FEED_ENUM."CAMERA MINIMIZE") -> ()  [unwired: 9 in, 2 out]
          }
        }
        n742 = case shown="True" w1112 {
          selector: w1112 -> [_ w1118]
          frame False {
          }
          frame True {
            n743 = Not(x=w1118) -> (.not. x?=w1117:bool)
            n744 = local write "CAMERA ROI MIN TEMP"(w1117) -> ()
            n745 = call "IMAGE ANALYSIS.vi"("Enum"=POST_ANALYSIS_ENUM."MINIMIZE UI") -> ()  [unwired: 9 in, 2 out]
          }
        }
        n746 = local write "CAMERA ROI MAX TEMP"(TRUE ("CAMERA ROI MAX TEMP")) -> ()
      }
      frame "Test Setup" {
        n747 = local read "LIVE FEED MIN TEMP"() -> (w1124:bool)
        n748 = local read "CAMERA ROI MIN TEMP"() -> (w1122:bool)
        n749 = local write "LIVE FEED MAX TEMP"(TRUE ("LIVE FEED MAX TEMP")) -> ()
        n750 = case shown="True" w1124 {
          selector: w1124 -> [_ w1131]
          frame False {
          }
          frame True {
            n751 = Not(x=w1131) -> (.not. x?=w1130:bool)
            n752 = local write "LIVE FEED MIN TEMP"(w1130) -> ()
            n753 = call "CAMERA LIVE FEED FGV.vi"("Enum - Menu"=CAMERA_LIVE_FEED_ENUM."CAMERA MINIMIZE") -> ()  [unwired: 9 in, 2 out]
          }
        }
        n754 = case shown="True" w1122 {
          selector: w1122 -> [_ w1128]
          frame False {
          }
          frame True {
            n755 = Not(x=w1128) -> (.not. x?=w1127:bool)
            n756 = local write "CAMERA ROI MIN TEMP"(w1127) -> ()
            n757 = call "IMAGE ANALYSIS.vi"("Enum"=POST_ANALYSIS_ENUM."MINIMIZE UI") -> ()  [unwired: 9 in, 2 out]
          }
        }
        n758 = local write "CAMERA ROI MAX TEMP"(TRUE ("CAMERA ROI MAX TEMP")) -> ()
      }
      frame "Acquire" {
        n759 = local read "LIVE FEED MIN TEMP"() -> (w1134:bool)
        n760 = local write "LIVE FEED MAX TEMP"(TRUE ("LIVE FEED MAX TEMP")) -> ()
        n761 = local read "CAMERA ROI MIN TEMP"() -> (w1132:bool)
        n762 = case shown="True" w1134 {
          selector: w1134 -> [_ w1141]
          frame False {
          }
          frame True {
            n763 = Not(x=w1141) -> (.not. x?=w1140:bool)
            n764 = local write "LIVE FEED MIN TEMP"(w1140) -> ()
            n765 = call "CAMERA LIVE FEED FGV.vi"("Enum - Menu"=CAMERA_LIVE_FEED_ENUM."CAMERA MINIMIZE") -> ()  [unwired: 9 in, 2 out]
          }
        }
        n766 = case shown="True" w1132 {
          selector: w1132 -> [_ w1138]
          frame False {
          }
          frame True {
            n767 = Not(x=w1138) -> (.not. x?=w1137:bool)
            n768 = local write "CAMERA ROI MIN TEMP"(w1137) -> ()
            n769 = call "IMAGE ANALYSIS.vi"("Enum"=POST_ANALYSIS_ENUM."MINIMIZE UI") -> ()  [unwired: 9 in, 2 out]
          }
        }
        n770 = local write "CAMERA ROI MAX TEMP"(TRUE ("CAMERA ROI MAX TEMP")) -> ()
      }
      frame "Adv Scar" {
        n771 = local read "CAMERA ROI MIN TEMP"() -> (w1142:bool)
        n772 = case shown="True" "LIVE FEED MAX TEMP" {
          selector: "LIVE FEED MAX TEMP" -> [_ w1163]
          frame False {
          }
          frame True {
            n773 = Not(x=w1163) -> (.not. x?=w1162:bool)
            n774 = local write "LIVE FEED MAX TEMP"(w1162) -> ()
            n775 = call "CAMERA LIVE FEED FGV.vi"("Enum - Menu"=CAMERA_LIVE_FEED_ENUM."CAMERA RESTORE") -> ("error out"=w1153:errorcluster)  [unwired: 9 in, 1 out]
            n776 = Type Cast(type=30, x=0) -> (*(type *) &x=w1157:i32)
            n777 = Add(x=w1157, y=48) -> (x+y=w1158:i32)
            n778 = call "CAMERA LIVE FEED FGV.vi"("Enum - Menu"=CAMERA_LIVE_FEED_ENUM."CAMERA MODE SET", "error in (no error)"=w1153, "CAMERA MODE"=w1158) -> ("error out"=w1150:errorcluster)  [unwired: 7 in, 1 out]
            n779 = call "CAMERA LIVE FEED FGV.vi"("Enum - Menu"=CAMERA_LIVE_FEED_ENUM."CAMERA GRAY", "error in (no error)"=w1150) -> ("error out"=w1149:errorcluster)  [unwired: 8 in, 1 out]
            n780 = call "LIST FILE NAMES.vi"("error in (no error)"=w1149) -> ("error out"=w1159:errorcluster, "filenames"=w1160:string[])  [unwired: 9 in]
            n781 = property on="FILE 3" class="CmbBox"(error in=w1159, "Strings[]"=w1160) -> ()  [unwired: 1 in, 2 out]
          }
        }
        n782 = case shown="True" w1142 {
          selector: w1142 -> [_ w1148]
          frame False {
          }
          frame True {
            n783 = Not(x=w1148) -> (.not. x?=w1147:bool)
            n784 = local write "CAMERA ROI MIN TEMP"(w1147) -> ()
            n785 = call "IMAGE ANALYSIS.vi"("Enum"=POST_ANALYSIS_ENUM."MINIMIZE UI") -> ()  [unwired: 9 in, 2 out]
          }
        }
        n786 = local write "CAMERA ROI MAX TEMP"(TRUE ("CAMERA ROI MAX TEMP")) -> ()
        "LIVE FEED MIN TEMP" <- TRUE ("LIVE FEED MIN TEMP")
      }
      frame "Adv Scar Report" {
        n787 = local read "CAMERA ROI MAX TEMP"() -> (w1164:bool)
        n788 = local read "LIVE FEED MIN TEMP"() -> (w1166:bool)
        n789 = local write "LIVE FEED MAX TEMP"(TRUE ("LIVE FEED MAX TEMP")) -> ()
        n790 = case shown="True" w1166 {
          selector: w1166 -> [_ w1175]
          frame False {
          }
          frame True {
            n791 = Not(x=w1175) -> (.not. x?=w1174:bool)
            n792 = local write "LIVE FEED MIN TEMP"(w1174) -> ()
            n793 = call "CAMERA LIVE FEED FGV.vi"("Enum - Menu"=CAMERA_LIVE_FEED_ENUM."CAMERA MINIMIZE") -> ()  [unwired: 9 in, 2 out]
          }
        }
        n794 = case shown="True" w1164 {
          selector: w1164 -> [_ w1172]
          frame False {
          }
          frame True {
            n795 = Not(x=w1172) -> (.not. x?=w1170:bool)
            n796 = local write "CAMERA ROI MAX TEMP"(w1170) -> ()
            n797 = call "IMAGE ANALYSIS.vi"("Enum"=POST_ANALYSIS_ENUM."SHOW UI") -> ("error out"=w1169:errorcluster)  [unwired: 9 in, 1 out]
            n798 = call "LIST FILE NAMES.vi"("error in (no error)"=w1169) -> ("filenames"=w1168:string[])  [unwired: 9 in, 1 out]
            n799 = property on="Test File List :" class="CmbBox"("Strings[]"=w1168) -> ()  [unwired: 2 in, 2 out]
          }
        }
        n800 = local write "CAMERA ROI MIN TEMP"(TRUE ("CAMERA ROI MIN TEMP")) -> ()
      }
      frame "Compare Files" {
        n801 = local read "LIVE FEED MIN TEMP"() -> (w1178:bool)
        n802 = local write "LIVE FEED MAX TEMP"(TRUE ("LIVE FEED MAX TEMP")) -> ()
        n803 = local read "CAMERA ROI MIN TEMP"() -> (w1176:bool)
        n804 = case shown="True" w1178 {
          selector: w1178 -> [_ w1185]
          frame False {
          }
          frame True {
            n805 = Not(x=w1185) -> (.not. x?=w1184:bool)
            n806 = local write "LIVE FEED MIN TEMP"(w1184) -> ()
            n807 = call "CAMERA LIVE FEED FGV.vi"("Enum - Menu"=CAMERA_LIVE_FEED_ENUM."CAMERA MINIMIZE") -> ()  [unwired: 9 in, 2 out]
          }
        }
        n808 = case shown="True" w1176 {
          selector: w1176 -> [_ w1182]
          frame False {
          }
